vi "4x7segment.vi"(11 "Numeric Control":dbl format="%#_13g") -> (3 "?":T7)   [LabVIEW 2019]
uses:
  4x7 segment controls/top-segment.ctl
  4x7 segment controls/left-segment.ctl
  4x7 segment controls/rigt-segment.ctl
  4x7 segment controls/mid-segment.ctl
  4x7 segment controls/bottom-segment.ctl
  4x7 segment controls/decimal.ctl
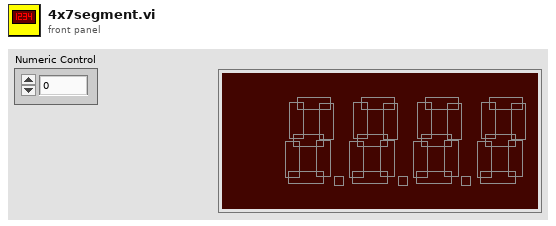
[diagram p1: front panel]
types:
  T1 = typedef "top-segment.ctl" = bool
  T2 = typedef "left-segment.ctl" = bool
  T3 = typedef "rigt-segment.ctl" = bool
  T4 = typedef "mid-segment.ctl" = bool
  T5 = typedef "bottom-segment.ctl" = bool
  T6 = typedef "decimal.ctl" = bool
  T7 = cluster{"1":cluster{"1":T1, "2":T2, "3":T3, "4":T4, "5":T2, "6":T3, "7":T5}, "2":cluster{"1":T1, "2":T2, "3":T3, "4":T4, "5":T2, "6":T3, "7":T5}, "3":cluster{"1":T1, "2":T2, "3":T3, "4":T4, "5":T2, "6":T3, "7":T5}, "4":cluster{"1":T1, "2":T2, "3":T3, "4":T4, "5":T2, "6":T3, "7":T5}, T6, T6, T6}
  T8 = cluster{"1":T1, "2":T2, "3":T3, "4":T4, "5":T2, "6":T3, "7":T5}
  T9 = cluster{"1":T1, "2":T2, "3":T3, "4":T4, "5":T2, "6":T3, "7":T5}[]
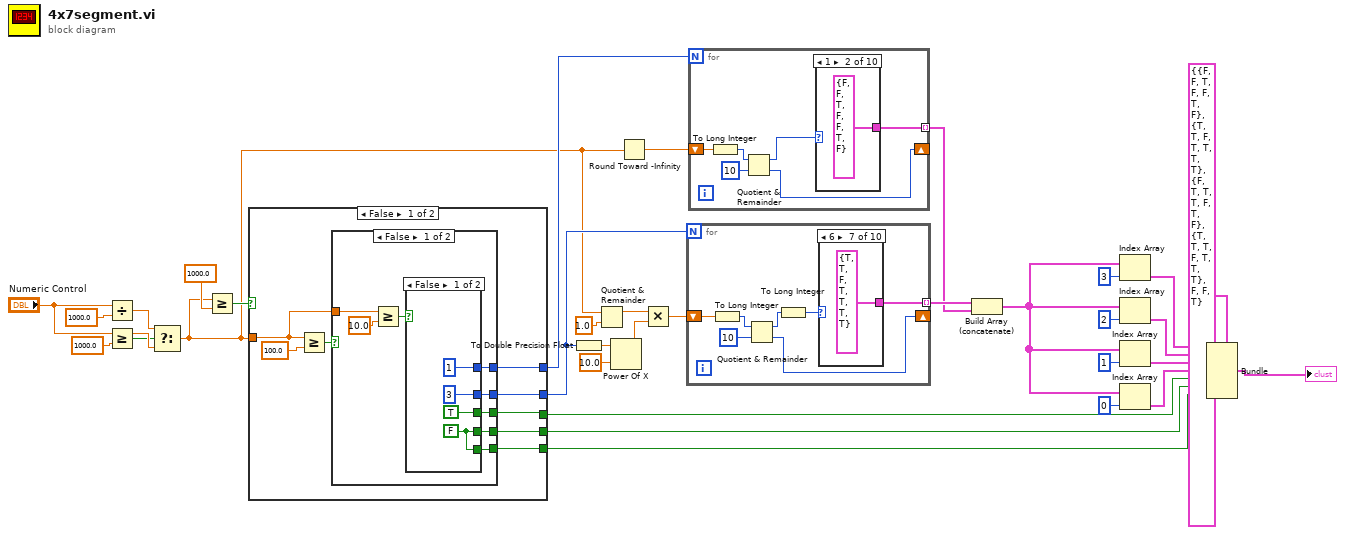
[diagram p0: block diagram]
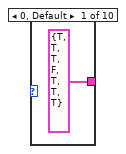
[diagram p2: hidden frame]
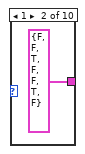
[diagram p3: hidden frame]
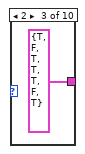
[diagram p4: hidden frame]
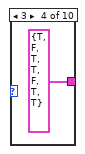
[diagram p5: hidden frame]
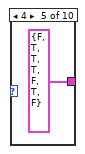
[diagram p6: hidden frame]
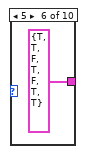
[diagram p7: hidden frame]
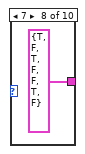
[diagram p8: hidden frame]
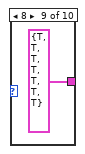
[diagram p9: hidden frame]
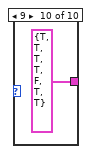
[diagram p10: hidden frame]
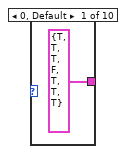
[diagram p11: hidden frame]
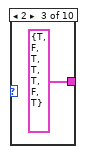
[diagram p12: hidden frame]
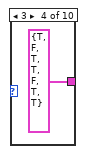
[diagram p13: hidden frame]
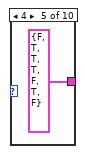
[diagram p14: hidden frame]
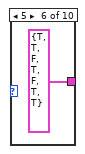
[diagram p15: hidden frame]
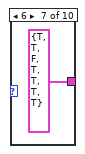
[diagram p16: hidden frame]
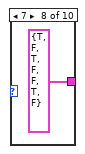
[diagram p17: hidden frame]
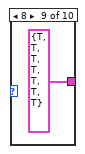
[diagram p18: hidden frame]
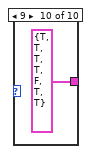
[diagram p19: hidden frame]
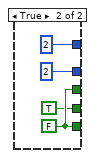
[diagram p20: hidden frame]
diagram:
  n1 = Divide(x="Numeric Control", y=1000.0) -> (x/y=w31:dbl)
  n2 = Greater Or Equal?(x="Numeric Control", y=1000.0) -> (x >= y?=w2:bool)
  n3 = Select(t=w31, s=w2, f="Numeric Control") -> (s? t:f=w4:dbl)
  n4 = Greater Or Equal?(x=w4, y=1000.0) -> (x >= y?=w7:bool)
  n5 = case shown="False" w7 {
    tunnel: [w37 w62] -> w22
    tunnel: [w36 w62] -> w21
    tunnel: [w38 w62] -> w20
    tunnel: w4 -> [w35 _]
    tunnel: [w39 4] -> w18
    tunnel: [w34 0] -> w11
    frame False {
      n6 = Greater Or Equal?(x=w35, y=100.0) -> (x >= y?=w40:bool)
      n7 = case shown="False" w40 {
        tunnel: [w43 3] -> w39
        tunnel: [w42 1] -> w34
        tunnel: [w46 T6 TRUE] -> w38
        tunnel: [w45 w58] -> w37
        tunnel: [w44 w58] -> w36
        tunnel: w35 -> [w49 _]
        frame False {
          n8 = Greater Or Equal?(x=w49, y=10.0) -> (x >= y?=w47:bool)
          n9 = case shown="False" w47 {
            tunnel: [w50 w57] -> w46
            tunnel: [T6 TRUE w57] -> w45
            tunnel: [w50 T6 TRUE] -> w44
            tunnel: [1 2] -> w43
            tunnel: [3 2] -> w42
            frame False {
              w50 = T6 FALSE
            }
            frame True {
              w57 = T6 FALSE
            }
          }
        }
        frame True {
          w58 = T6 FALSE
        }
      }
    }
    frame True {
      w62 = T6 FALSE
    }
  }
  n10 = To Double Precision Float(number=w11) -> (double precision float=w13:dbl)
  n11 = Quotient & Remainder(x=w4, y=1.0) -> (x-y*floor(x/y)=w16:dbl)  [unwired: 1 out]
  n12 = Power Of X(1:10.0 ("x"), 2:w13) -> (0:w15:dbl)
  n13 = Round Toward -Infinity(1:w4) -> (0:w5:dbl)
  n14 = Multiply(x=w16, y=w15) -> (x*y=w12:dbl)
  n15 = for {
    N: w11 -> [_]
    shift-right: [w71] -> _
    shift-left: w12 -> [w67]
    tunnel: [w68] -> w9 mode=indexing
    n16 = To Long Integer(number=w67) -> (32bit integer=w66:i32)
    n17 = Quotient & Remainder(x=w66, y=10) -> (x-y*floor(x/y)=w70:i32, floor(x/y)=w71:i32)
    n18 = To Long Integer(number=w70) -> (32bit integer=w69:i32)
    n19 = case shown="6" w69 {
      tunnel: [T8 {"1"=TRUE, "2"=TRUE, "3"=TRUE, "4"=FALSE, "5"=TRUE, "6"=TRUE, "7"=TRUE} ("1") T8 {"1"=FALSE, "2"=FALSE, "3"=TRUE, "4"=FALSE, "5"=FALSE, "6"=TRUE, "7"=FALSE} ("1") T8 {"1"=TRUE, "2"=FALSE, "3"=TRUE, "4"=TRUE, "5"=TRUE, "6"=FALSE, "7"=TRUE} ("1") T8 {"1"=TRUE, "2"=FALSE, "3"=TRUE, "4"=TRUE, "5"=FALSE, "6"=TRUE, "7"=TRUE} ("1") T8 {"1"=FALSE, "2"=TRUE, "3"=TRUE, "4"=TRUE, "5"=FALSE, "6"=TRUE, "7"=FALSE} ("1") T8 {"1"=TRUE, "2"=TRUE, "3"=FALSE, "4"=TRUE, "5"=FALSE, "6"=TRUE, "7"=TRUE} ("1") T8 {"1"=TRUE, "2"=TRUE, "3"=FALSE, "4"=TRUE, "5"=TRUE, "6"=TRUE, "7"=TRUE} ("1") T8 {"1"=TRUE, "2"=FALSE, "3"=TRUE, "4"=FALSE, "5"=FALSE, "6"=TRUE, "7"=FALSE} ("1") T8 {"1"=TRUE, "2"=TRUE, "3"=TRUE, "4"=TRUE, "5"=TRUE, "6"=TRUE, "7"=TRUE} ("1") T8 {"1"=TRUE, "2"=TRUE, "3"=TRUE, "4"=TRUE, "5"=FALSE, "6"=TRUE, "7"=TRUE} ("1")] -> w68
      frame 0, Default {
      }
      frame 1 {
      }
      frame 2 {
      }
      frame 3 {
      }
      frame 4 {
      }
      frame 5 {
      }
      frame 6 {
      }
      frame 7 {
      }
      frame 8 {
      }
      frame 9 {
      }
    }
  }
  n20 = for {
    N: w18 -> [_]
    shift-right: [w87] -> _
    shift-left: w5 -> [w85]
    tunnel: [w86] -> w8 mode=indexing
    n21 = To Long Integer(number=w85) -> (32bit integer=w84:i32)
    n22 = Quotient & Remainder(x=w84, y=10) -> (x-y*floor(x/y)=w83:i32, floor(x/y)=w87:i32)
    n23 = case shown="1" w83 {
      tunnel: [T8 {"1"=TRUE, "2"=TRUE, "3"=TRUE, "4"=FALSE, "5"=TRUE, "6"=TRUE, "7"=TRUE} ("1") T8 {"1"=FALSE, "2"=FALSE, "3"=TRUE, "4"=FALSE, "5"=FALSE, "6"=TRUE, "7"=FALSE} ("1") T8 {"1"=TRUE, "2"=FALSE, "3"=TRUE, "4"=TRUE, "5"=TRUE, "6"=FALSE, "7"=TRUE} ("1") T8 {"1"=TRUE, "2"=FALSE, "3"=TRUE, "4"=TRUE, "5"=FALSE, "6"=TRUE, "7"=TRUE} ("1") T8 {"1"=FALSE, "2"=TRUE, "3"=TRUE, "4"=TRUE, "5"=FALSE, "6"=TRUE, "7"=FALSE} ("1") T8 {"1"=TRUE, "2"=TRUE, "3"=FALSE, "4"=TRUE, "5"=FALSE, "6"=TRUE, "7"=TRUE} ("1") T8 {"1"=TRUE, "2"=TRUE, "3"=FALSE, "4"=TRUE, "5"=TRUE, "6"=TRUE, "7"=TRUE} ("1") T8 {"1"=TRUE, "2"=FALSE, "3"=TRUE, "4"=FALSE, "5"=FALSE, "6"=TRUE, "7"=FALSE} ("1") T8 {"1"=TRUE, "2"=TRUE, "3"=TRUE, "4"=TRUE, "5"=TRUE, "6"=TRUE, "7"=TRUE} ("1") T8 {"1"=TRUE, "2"=TRUE, "3"=TRUE, "4"=TRUE, "5"=FALSE, "6"=TRUE, "7"=TRUE} ("1")] -> w86
      frame 0, Default {
      }
      frame 1 {
      }
      frame 2 {
      }
      frame 3 {
      }
      frame 4 {
      }
      frame 5 {
      }
      frame 6 {
      }
      frame 7 {
      }
      frame 8 {
      }
      frame 9 {
      }
    }
  }
  n24 = Build Array (concatenate)(w9, w8) -> (w10:T9)
  n25 = Index Array(array=w10, index=3) -> (element=w26:T8)
  n26 = Index Array(array=w10, index=2) -> (element=w25:T8)
  n27 = Index Array(array=w10, index=1) -> (element=w24:T8)
  n28 = Index Array(array=w10, index=0) -> (element=w23:T8)
  n29 = Bundle(cluster=T7 {"1"={"1"=FALSE, "2"=FALSE, "3"=TRUE, "4"=FALSE, "5"=FALSE, "6"=TRUE, "7"=FALSE}, "2"={"1"=TRUE, "2"=TRUE, "3"=FALSE, "4"=TRUE, "5"=TRUE, "6"=TRUE, "7"=TRUE}, "3"={"1"=FALSE, "2"=TRUE, "3"=TRUE, "4"=TRUE, "5"=FALSE, "6"=TRUE, "7"=FALSE}, "4"={"1"=TRUE, "2"=TRUE, "3"=TRUE, "4"=FALSE, "5"=TRUE, "6"=TRUE, "7"=TRUE}, FALSE, FALSE, TRUE}, "1"=w26, "2"=w25, "3"=w24, "4"=w23, w22, w21, w20) -> (→"?":T7)
